vi "DG GUI Measurement setup.vi"(9 "DG measurement":T1={"Signal frequencies (Hz)"=[1000.0], "Signal amplitudes (V)"=[0.707], "Sampling frequencies (Hz)"=[10000000.0], "Record lengths (multiples of periods)"=[10000.0], "Calculate results"=FALSE, "Algorithm"="TWM-PJVSSubS", "TWM data directories"=[], "TWM data directories relative"=[], "PJVS frequencies (Hz)"=[1000.0], "PJVS reference voltages array of vector cluster"=[], "Requested PJVS steps"=[20], "Data folder"=path "", "Rs"=0, "Re"=0, "Settle down after PJVS change (s)"=1.0, "Switch position"=0.0, "PJVS amplitudes (Hz)"=[1000.0]} {"PJVS amplitudes (Hz)" format="%#_3p"; "PJVS reference voltages array of vector cluster"."PJVS reference voltages vector" format="%#_3p"; "PJVS frequencies (Hz)" format="%#_3p"; "Record lengths (multiples of periods)" format="%#_3p"; "Sampling frequencies (Hz)" format="%#_3p"; "Signal amplitudes (V)" format="%#_3p"; "Signal frequencies (Hz)" format="%#_3p"}) -> (3 "DG measurement out":T1={"Signal frequencies (Hz)"=[1000.0], "Signal amplitudes (V)"=[0.707], "Sampling frequencies (Hz)"=[10000000.0], "Record lengths (multiples of periods)"=[10000.0], "Calculate results"=FALSE, "Algorithm"="TWM-PJVSSubS", "TWM data directories"=[], "TWM data directories relative"=[], "PJVS frequencies (Hz)"=[1000.0], "PJVS reference voltages array of vector cluster"=[], "Requested PJVS steps"=[20], "Data folder"=path "", "Rs"=0, "Re"=0, "Settle down after PJVS change (s)"=1.0, "Switch position"=0.0, "PJVS amplitudes (Hz)"=[1000.0]} {"PJVS amplitudes (Hz)" format="%#_3p"; "PJVS reference voltages array of vector cluster"."PJVS reference voltages vector" format="%#_3p"; "PJVS frequencies (Hz)" format="%#_3p"; "Record lengths (multiples of periods)" format="%#_3p"; "Sampling frequencies (Hz)" format="%#_3p"; "Signal amplitudes (V)" format="%#_3p"; "Signal frequencies (Hz)" format="%#_3p"})   [LabVIEW 2020]
doc: "GUI to setup parameters of the digitizer gain calibration mesurement procedure."
uses:
  SS Measurement/Type definitions/SS measurement.ctl
  DG Measurement/DG measurement.ctl
  <vilib>/Utility/error.llb/Error Cluster From Error Code.vi
  <vilib>/ErrorRing/Error Ring.xnode
  external libraries/varilib/varilib.lvlib
panel:
  in  "Signal amplitude (V)":dbl=1.0 format="%#_13g"
  in  "Switch position":bool
  in  "Re":i32 min=0 step=1
  in  "Rs":i32 min=0 step=1
  out "No of samples":dbl format="%#_6p"
  out "Sampling time (s)":dbl
  out "DG error":string="!"
  out "Is coherent":string="!"
  in  "Data folder":path caption="Save data to folder:"
  in  "Requested PJVS steps":u32
  out "Requested PJVS steps out":u32[](array[numeric])
  in  "PJVS frequency (Hz)":dbl
  out "PJVS frequencies (Hz) out":dbl[](array[numeric])
  in  "Record length (multiple of period)":dbl
  out "SS measurement out":T2={"Signal frequencies (Hz)"=[1000.0], "Signal amplitudes (V)"=[0.707], "Sampling frequencies (Hz)"=[10000000.0], "Record lengths (multiples of periods)"=[10000.0], "Calculate results"=FALSE, "Algorithm"="TWM-WFFT", "TWM data directories"=[], "TWM data directories relative"=[], "Settle down after AC source change (s)"=1.0, "PJVS frequencies (Hz)"=[1000.0], "PJVS reference voltages array of vector cluster"=[{"PJVS reference voltages vector"=[]}], "Requested PJVS steps"=[20], "Measure CE"=FALSE, "Measure CE before"=FALSE, "Measure CE after"=FALSE, "Single point CE measurement"=FALSE, "original CE template path"=path "", "new CE template path before SS"=path "", "new CE template path before SS relative"=path "", "new CE template path after SS"=path "", "new CE template path after SS relative"=path "", "original CE fit path"=path "", "new CE fit path before SS"=path "", "new CE fit path before SS relative"=path "", "new CE fit path after SS"=path "", "new CE fit path after SS relative"=path "", "Measure digitizer gain"=FALSE, "Measure digitizer gain before"=FALSE, "Measure digitizer gain after"=FALSE, "Digitizer gain"=0.0, "Data folder"=path "", "FR fit path"=path "", "new FR fit path relative"=path "", "Rs"=0, "Re"=0, "SS measurement info files"=[]} {"PJVS reference voltages array of vector cluster"."PJVS reference voltages vector" format="%#_3p"; "PJVS frequencies (Hz)" format="%#_3p"; "Record lengths (multiples of periods)" format="%#_3p"; "Sampling frequencies (Hz)" format="%#_3p"; "Signal amplitudes (V)" format="%#_3p"; "Signal frequencies (Hz)" format="%#_3p"}
  in  "SS measurement":T2={"Signal frequencies (Hz)"=[1000.0], "Signal amplitudes (V)"=[0.707], "Sampling frequencies (Hz)"=[10000000.0], "Record lengths (multiples of periods)"=[10000.0], "Calculate results"=FALSE, "Algorithm"="TWM-WFFT", "TWM data directories"=[], "TWM data directories relative"=[], "Settle down after AC source change (s)"=1.0, "PJVS frequencies (Hz)"=[1000.0], "PJVS reference voltages array of vector cluster"=[{"PJVS reference voltages vector"=[]}], "Requested PJVS steps"=[20], "Measure CE"=FALSE, "Measure CE before"=FALSE, "Measure CE after"=FALSE, "Single point CE measurement"=FALSE, "original CE template path"=path "", "new CE template path before SS"=path "", "new CE template path before SS relative"=path "", "new CE template path after SS"=path "", "new CE template path after SS relative"=path "", "original CE fit path"=path "", "new CE fit path before SS"=path "", "new CE fit path before SS relative"=path "", "new CE fit path after SS"=path "", "new CE fit path after SS relative"=path "", "Measure digitizer gain"=FALSE, "Measure digitizer gain before"=FALSE, "Measure digitizer gain after"=FALSE, "Digitizer gain"=0.0, "Data folder"=path "", "FR fit path"=path "", "new FR fit path relative"=path "", "Rs"=0, "Re"=0, "SS measurement info files"=[]} {"PJVS reference voltages array of vector cluster"."PJVS reference voltages vector" format="%#_3p"; "PJVS frequencies (Hz)" format="%#_3p"; "Record lengths (multiples of periods)" format="%#_3p"; "Sampling frequencies (Hz)" format="%#_3p"; "Signal amplitudes (V)" format="%#_3p"; "Signal frequencies (Hz)" format="%#_3p"}
  in  "Calculate results":bool
  in  "Algorithm":string
  out "Signal amplitudes (V) out":dbl[](array[numeric])
  out "Record lengths (multiples of period)":dbl[](array[numeric])
  out "Sampling frequencies (Hz) out":dbl[](array[numeric])
  in  "Settle down after PJVS change (s)":dbl=1.0 format="%#_13g"
  in  "Sampling frequency (Hz)":dbl=10000000.0 format="%#_13p"
  in  "show connections":bool
  out "gui_elements":refnum<vi>[](array[refnum])
  in  "save_and_quit":bool
  in  "cancel":bool
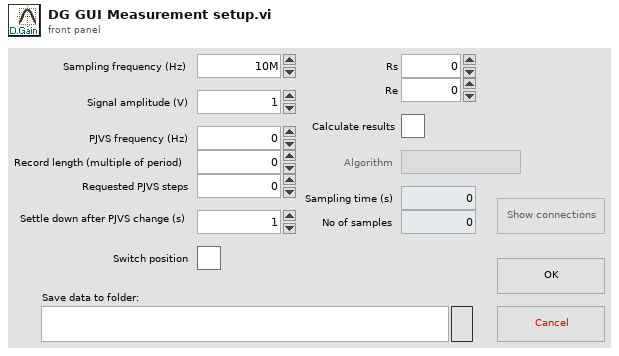
[diagram p1: front panel]
types:
  T1 = typedef "DG measurement.ctl" = cluster{"Signal frequencies (Hz)":dbl[], "Signal amplitudes (V)":dbl[], "Sampling frequencies (Hz)":dbl[], "Record lengths (multiples of periods)":dbl[], "Calculate results":bool, "Algorithm":string, "TWM data directories":path[], "TWM data directories relative":path[], "PJVS frequencies (Hz)":dbl[], "PJVS reference voltages array of vector cluster":cluster{"PJVS reference voltages vector":dbl[]}[], "Requested PJVS steps":u32[], "Data folder":path, "Rs":i32, "Re":i32, "Settle down after PJVS change (s)":dbl, "Switch position":dbl, "PJVS amplitudes (Hz)":dbl[]}
  T2 = typedef "SS measurement.ctl" = cluster{"Signal frequencies (Hz)":dbl[], "Signal amplitudes (V)":dbl[], "Sampling frequencies (Hz)":dbl[], "Record lengths (multiples of periods)":dbl[], "Calculate results":bool, "Algorithm":string, "TWM data directories":path[], "TWM data directories relative":path[], "Settle down after AC source change (s)":dbl, "PJVS frequencies (Hz)":dbl[], "PJVS reference voltages array of vector cluster":cluster{"PJVS reference voltages vector":dbl[]}[], "Requested PJVS steps":u32[], "Measure CE":bool, "Measure CE before":bool, "Measure CE after":bool, "Single point CE measurement":bool, "original CE template path":path, "new CE template path before SS":path, "new CE template path before SS relative":path, "new CE template path after SS":path, "new CE template path after SS relative":path, "original CE fit path":path, "new CE fit path before SS":path, "new CE fit path before SS relative":path, "new CE fit path after SS":path, "new CE fit path after SS relative":path, "Measure digitizer gain":bool, "Measure digitizer gain before":bool, "Measure digitizer gain after":bool, "Digitizer gain":dbl, "Data folder":path, "FR fit path":path, "new FR fit path relative":path, "Rs":i32, "Re":i32, "SS measurement info files":path[]}
  T3 = enum32{"Bad", "Idle", "Run top level", "Running"}
  T4 = cluster{"PJVS reference voltages vector":dbl[]}[]
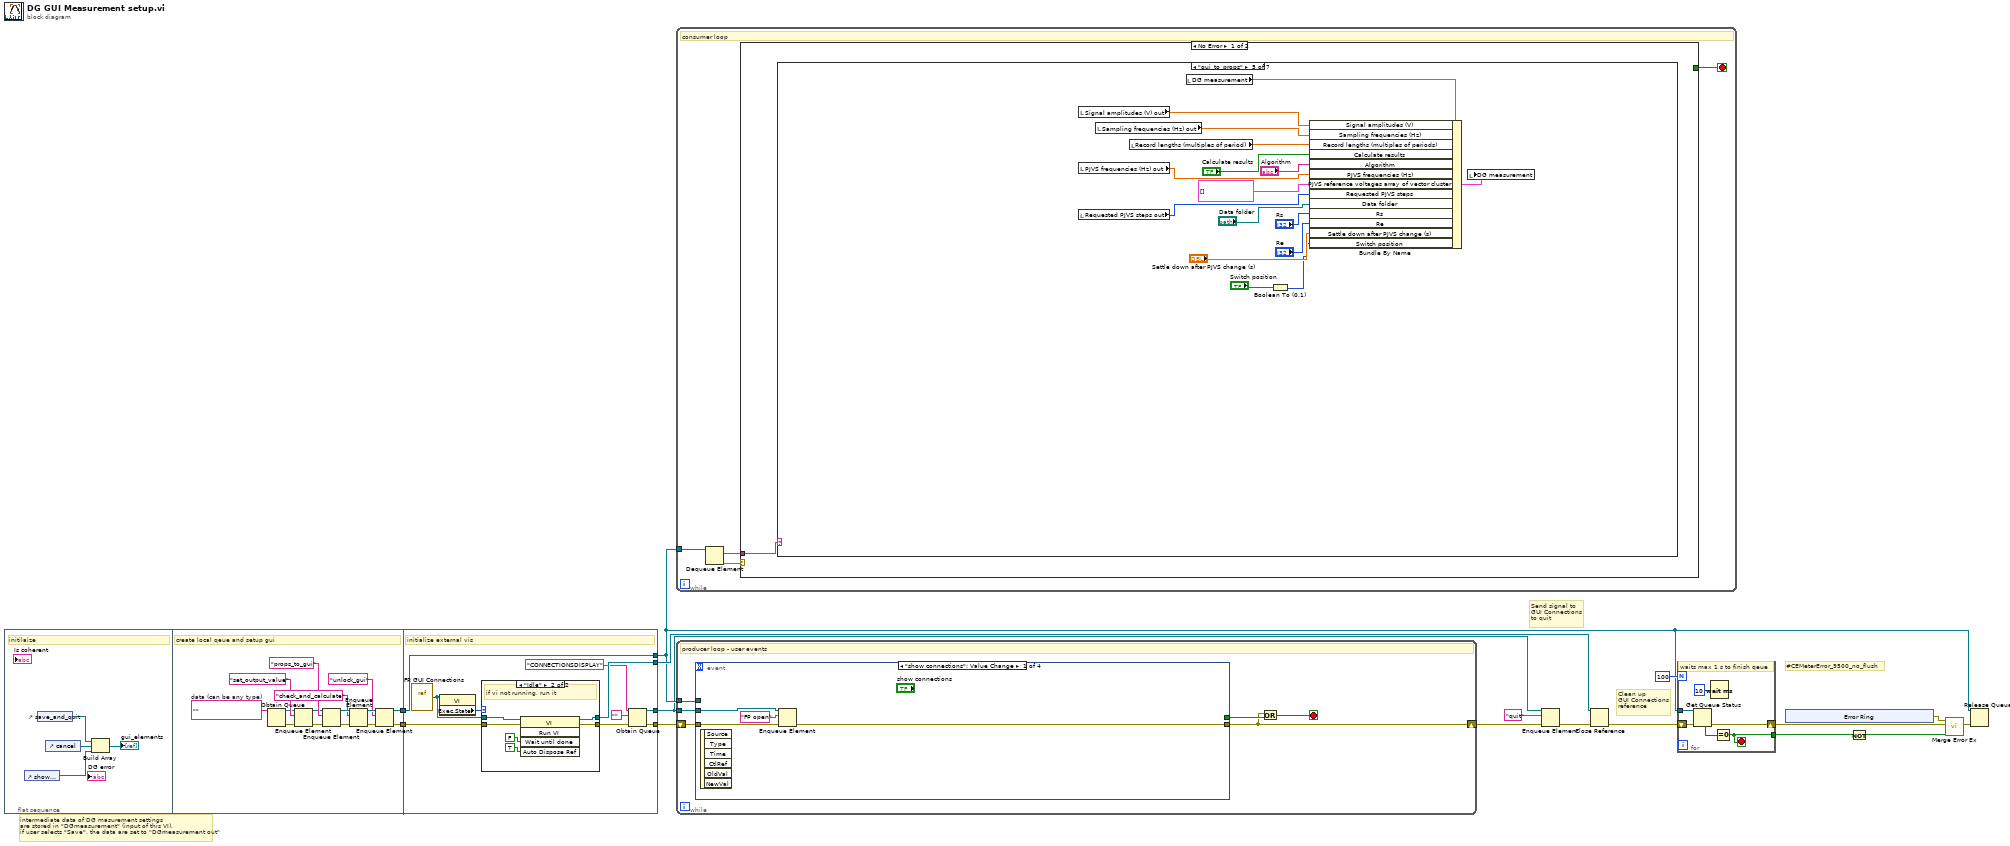
[diagram p0: block diagram]
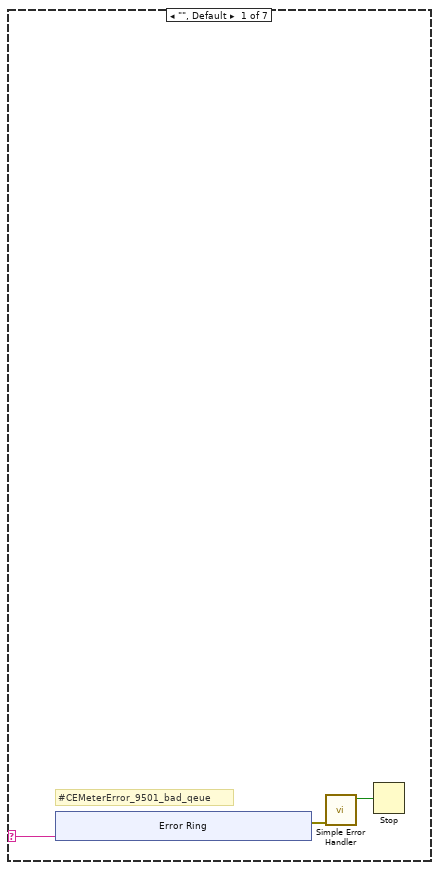
[diagram p3: hidden frame]
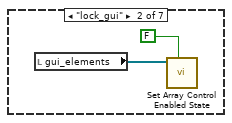
[diagram p4: hidden frame]
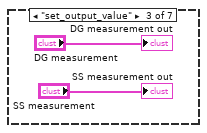
[diagram p5: hidden frame]
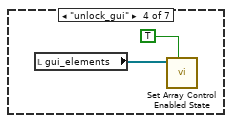
[diagram p6: hidden frame]
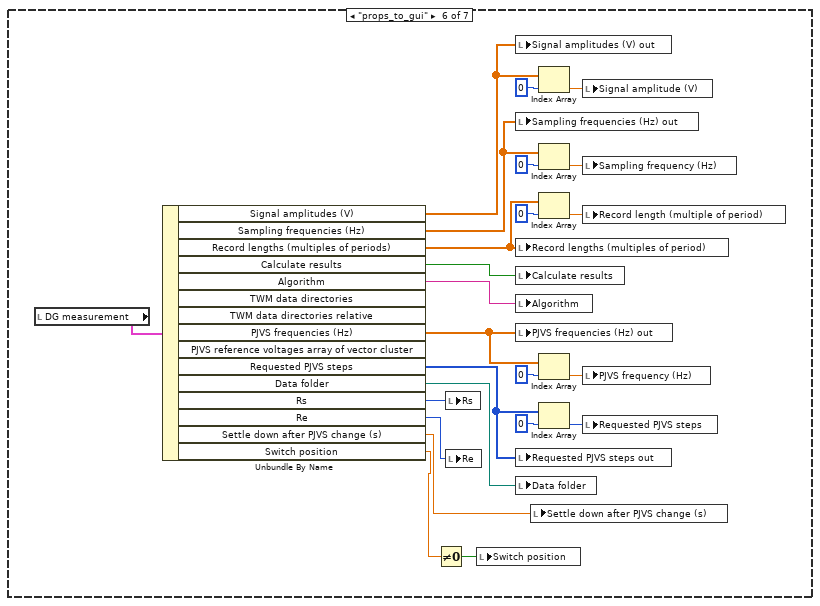
[diagram p7: hidden frame]
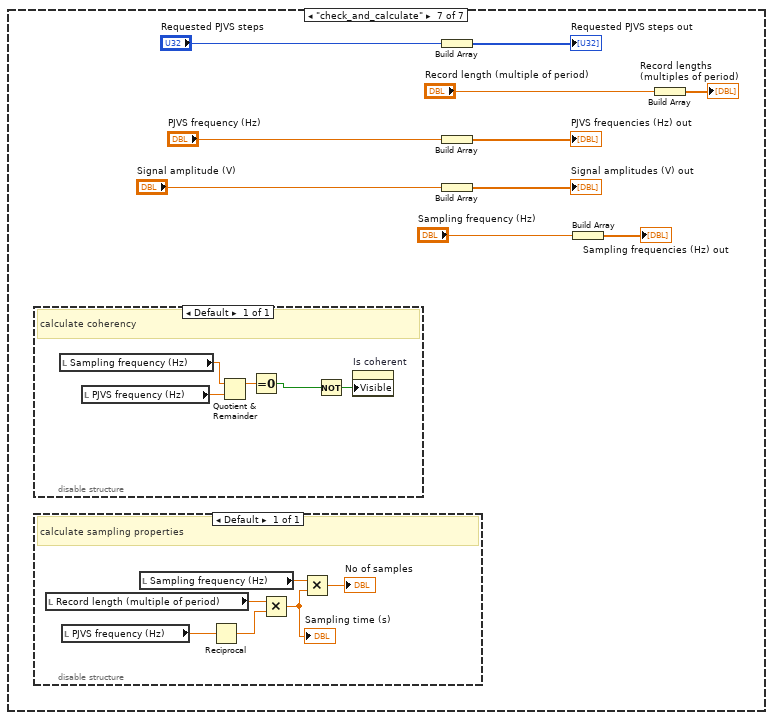
[diagram p8: hidden frame]
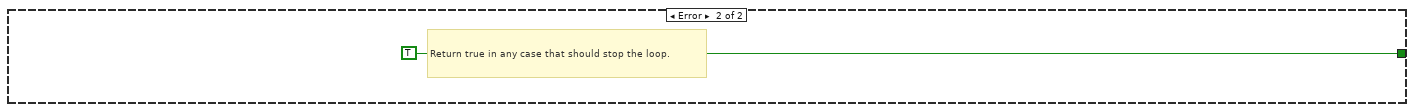
[diagram p9: hidden frame]
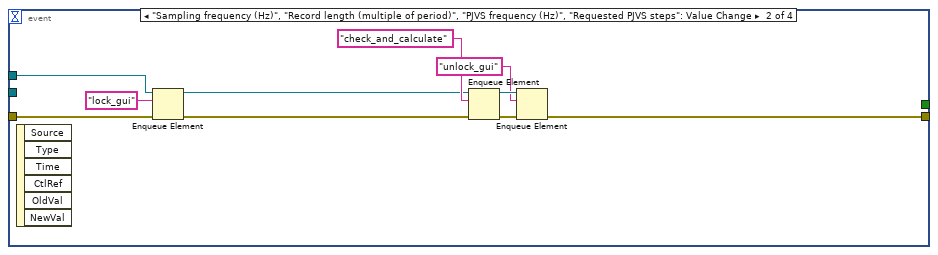
[diagram p10: hidden frame]
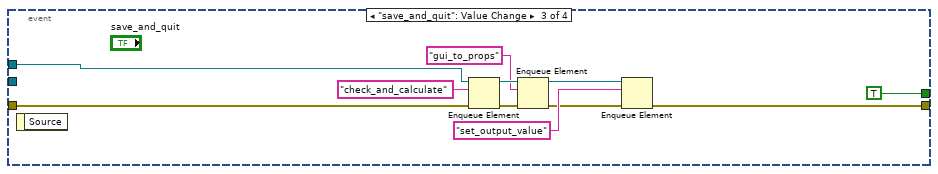
[diagram p11: hidden frame]
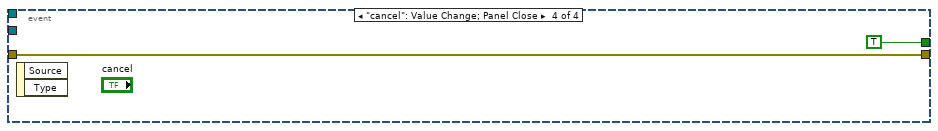
[diagram p12: hidden frame]
diagram:
  # "intermediate data of DG masurement settings\nare stored in \"DGmeasurement\" (input of this VI),\nif user selects \"Save\", the data are set to \"DGmeasurement out\""
  # "Send signal to\nGUI Connections\nto quit"
  # "Clean up\nGUI Connections\nreference"
  # "#CEMeterError_9500_no_flush"
  n1 = flat-sequence {
    tunnel: [w25] -> w9
    tunnel: [w24] -> w1
    tunnel: [w41] -> w10
    tunnel: [w45] -> w4
    tunnel: w9 -> [w44]
    tunnel: [w42] -> w3
    tunnel: [w43] -> w6
    tunnel: w1 -> [w45]
    frame #0 {
      # "initilaize"
      n2 = control-ref of="show connections"() -> (w17:refnum<vi>)
      n3 = control-ref of="save_and_quit"() -> (w20:refnum<vi>)
      n4 = control-ref of="cancel"() -> (w19:refnum<vi>)
      n5 = Build Array(w20, w19, w17) -> (→"gui_elements":refnum<vi>[])
    }
    frame #1 {
      w34 = ""  # data (can be any type)
      # "create local qeue and setup gui"
      n6 = Obtain Queue(element data type=w34) -> (queue out=w27:refnum<queue>, error out=w26:errorcluster)  [unwired: 4 in, 1 out]
      n7 = Enqueue Element(queue=w27, element="set_output_value", error in (no error)=w26) -> (queue out=w29:refnum<queue>, error out=w28:errorcluster)  [unwired: 1 in, 1 out]
      n8 = Enqueue Element(queue=w29, element="props_to_gui", error in (no error)=w28) -> (queue out=w32:refnum<queue>, error out=w33:errorcluster)  [unwired: 1 in, 1 out]
      n9 = Enqueue Element(queue=w32, element="check_and_calculate", error in (no error)=w33) -> (queue out=w23:refnum<queue>, error out=w22:errorcluster)  [unwired: 1 in, 1 out]
      n10 = Enqueue Element(queue=w23, element="unlock_gui", error in (no error)=w22) -> (queue out=w24:refnum<queue>, error out=w25:errorcluster)  [unwired: 1 in, 1 out]
    }
    frame #2 {
      # "initialize external vis"
      n11 = vi-ref "FR GUI Connections.vi"() -> (w39:refnum<vi>)
      n12 = property class="VI"(reference=w39) -> ("Exec.State"=w40:T3)  [unwired: 1 in, 2 out]
      n13 = case shown="\"Idle\"" w40 {
        tunnel: [w46 w53] -> w36
        tunnel: w44 -> [w46 w50]
        tunnel: [w47 w49] -> w43
        tunnel: w39 -> [w47 w48]
        frame "Bad", Default {
        }
        frame "Idle" {
          # "if vi not running, run it"
          n14 = invoke class="VI" method="Run VI"(reference=w48, error in=w50, "Wait until done"=FALSE ("Wait Until Done"), "Auto Dispose Ref"=TRUE ("Wait Until Done")) -> (reference out=w49:refnum<vi>, error out=w53:errorcluster)  [unwired: 1 in, 3 out]
        }
      }
      n15 = Obtain Queue(name (unnamed)="CONNECTIONSDISPLAY", element data type="", error in (no error)=w36) -> (queue out=w42:refnum<queue>, error out=w41:errorcluster)  [unwired: 2 in, 1 out]
    }
  }
  n16 = while {
    tunnel: w4 -> [w57]
    stop <- w54 stop-if-true
    # "consumer loop"
    n17 = Dequeue Element(queue=w57) -> (element=w55:string, error out=w56:errorcluster)  [unwired: 2 in, 2 out]
    n18 = case shown="No Error" w56 {
      tunnel: w55 -> [w58 _]
      tunnel: [_ TRUE] -> w54
      frame No Error {
        n19 = case shown="\"gui_to_props\"" w58 {
          selector: w58 -> [w59 _ _ _ _ _ _]
          frame "", Default {
            # "#CEMeterError_9501_bad_qeue"
            n20 = xnode "Error Ring"("parameter 0"=w59) -> ("error out"=w61:errorcluster)
            n21 = call <vilib>:"Simple Error Handler.vi"("error in (no error)"=w61) -> ("error?"=w60:bool)  [unwired: 4 in, 4 out]
            n22 = Stop(stop? (T)=w60) -> ()
          }
          frame "lock_gui" {
            n23 = local read "gui_elements"() -> (w70:refnum<vi>[])
            n24 = call "Set Array Control Enabled State.vi"("enabled (T)"=FALSE, "reference array in"=w70) -> ()  [unwired: 8 in, 2 out]
          }
          frame "set_output_value" {
            "SS measurement out" <- "SS measurement"
            "DG measurement out" <- "DG measurement"
          }
          frame "unlock_gui" {
            n25 = local read "gui_elements"() -> (w74:refnum<vi>[])
            n26 = call "Set Array Control Enabled State.vi"("enabled (T)"=TRUE, "reference array in"=w74) -> ()  [unwired: 8 in, 2 out]
          }
          frame "gui_to_props" {
            n27 = local read "Signal amplitudes (V) out"() -> (w86:dbl[])
            n28 = local read "PJVS frequencies (Hz) out"() -> (w81:dbl[])
            n29 = local read "Requested PJVS steps out"() -> (w79:u32[])
            n30 = local read "Sampling frequencies (Hz) out"() -> (w85:dbl[])
            n31 = local read "Record lengths (multiples of period)"() -> (w84:dbl[])
            n32 = local read "DG measurement"() -> (w90:T1)
            n33 = Boolean To (0,1)(Boolean="Switch position") -> (0, 1=w76:i16)
            n34 = Bundle By Name(cluster=w90, "Signal amplitudes (V)"=w86, "Sampling frequencies (Hz)"=w85, "Record lengths (multiples of periods)"=w84, "Calculate results"="Calculate results", "Algorithm"="Algorithm", "PJVS frequencies (Hz)"=w81, "PJVS reference voltages array of vector cluster"=T4 [], "Requested PJVS steps"=w79, "Data folder"="Data folder", "Rs"="Rs", "Re"="Re", "Settle down after PJVS change (s)"="Settle down after PJVS change (s)", "Switch position"=w76) -> (w89:T1)
            n35 = local write "DG measurement"(w89) -> ()
          }
          frame "props_to_gui" {
            n36 = local read "DG measurement"() -> (w104:T1)
            n37 = Unbundle By Name(w104) -> ("Signal amplitudes (V)"=w93:dbl[], "Sampling frequencies (Hz)"=w94:dbl[], "Record lengths (multiples of periods)"=w95:dbl[], "Calculate results"=w96:bool, "Algorithm"=w97:string, "PJVS frequencies (Hz)"=w98:dbl[], "Requested PJVS steps"=w99:u32[], "Data folder"=w100:path, "Rs"=w101:i32, "Re"=w102:i32, "Settle down after PJVS change (s)"=w103:dbl, "Switch position"=w92:dbl)  [unwired: 3 out]
            n38 = Not Equal To 0?(x=w92) -> (x != 0?=w91:bool)
            n39 = local write "Rs"(w101) -> ()
            n40 = local write "Re"(w102) -> ()
            n41 = local write "Switch position"(w91) -> ()
            n42 = local write "Signal amplitudes (V) out"(w93) -> ()
            n43 = local write "Sampling frequencies (Hz) out"(w94) -> ()
            n44 = local write "Record lengths (multiples of period)"(w95) -> ()
            n45 = local write "Calculate results"(w96) -> ()
            n46 = local write "Algorithm"(w97) -> ()
            n47 = local write "PJVS frequencies (Hz) out"(w98) -> ()
            n48 = local write "Requested PJVS steps out"(w99) -> ()
            n49 = local write "Data folder"(w100) -> ()
            n50 = local write "Settle down after PJVS change (s)"(w103) -> ()
            n51 = Index Array(array=w93, index=0) -> (element=w114:dbl)
            n52 = Index Array(array=w94, index=0) -> (element=w111:dbl)
            n53 = Index Array(array=w95, index=0) -> (element=w109:dbl)
            n54 = Index Array(array=w98, index=0) -> (element=w105:dbl)
            n55 = Index Array(array=w99, index=0) -> (element=w106:u32)
            n56 = local write "Signal amplitude (V)"(w114) -> ()
            n57 = local write "Sampling frequency (Hz)"(w111) -> ()
            n58 = local write "Record length (multiple of period)"(w109) -> ()
            n59 = local write "PJVS frequency (Hz)"(w105) -> ()
            n60 = local write "Requested PJVS steps"(w106) -> ()
          }
          frame "check_and_calculate" {
            n61 = disable-structure shown="Default" {
              frame Enabled {
                # "calculate coherency"
                n62 = local read "Sampling frequency (Hz)"() -> (w135:dbl)
                n63 = local read "PJVS frequency (Hz)"() -> (w134:dbl)
                n64 = Quotient & Remainder(x=w135, y=w134) -> (x-y*floor(x/y)=w133:dbl)  [unwired: 1 out]
                n65 = Equal To 0?(x=w133) -> (x = 0?=w131:bool)
                n66 = Not(x=w131) -> (.not. x?=w132:bool)
                n67 = property on="Is coherent" class="Str"("Visible"=w132) -> ()  [unwired: 2 in, 2 out]
              }
            }
            n68 = disable-structure shown="Default" {
              frame Enabled {
                # "calculate sampling properties"
                n69 = local read "Record length (multiple of period)"() -> (w128:dbl)
                n70 = local read "PJVS frequency (Hz)"() -> (w130:dbl)
                n71 = local read "Sampling frequency (Hz)"() -> (w127:dbl)
                n72 = Reciprocal(x=w130) -> (1/x=w129:dbl)
                n73 = Multiply(x=w128, y=w129) -> (x*y=w125:dbl)
                "Sampling time (s)" <- w125
                n74 = Multiply(x=w127, y=w125) -> (x*y=→"No of samples":dbl)
              }
            }
            n75 = Build Array("Requested PJVS steps") -> (→"Requested PJVS steps out":u32[])
            n76 = Build Array("PJVS frequency (Hz)") -> (→"PJVS frequencies (Hz) out":dbl[])
            n77 = Build Array("Signal amplitude (V)") -> (→"Signal amplitudes (V) out":dbl[])
            n78 = Build Array("Sampling frequency (Hz)") -> (→"Sampling frequencies (Hz) out":dbl[])
            n79 = Build Array("Record length (multiple of period)") -> (→"Record lengths (multiples of period)":dbl[])
          }
        }
      }
      frame Error {
        # "Return true in any case that should stop the loop."
      }
    }
  }
  n80 = while {
    shift-right: [w138] -> w5
    shift-left: w10 -> [w141]
    tunnel: w4 -> [w142]
    tunnel: w3 -> [w137]
    stop <- w139 stop-if-true
    # "producer loop - user events"
    n81 = event shown="[0] \"show connections\": Value Change" {
      selector: _ -> [_ _ _ _]
      dyn-events: _ -> [_ _ _ _]
      timeout: _ -> [_ _ _ _]
      tunnel: w142 -> [_ w155 w166 _]
      tunnel: w141 -> [w145 w148 w165 w168]
      tunnel: [w144 w147 w164 w168] -> w138
      tunnel: [_ _ TRUE ("cancel") TRUE ("cancel")] -> w140
      tunnel: w137 -> [w143 _ _ _]
      event "show connections": Value Change {
        n82 = event-data() -> ()  [unwired: 1 in, 6 out]
        n83 = Enqueue Element(queue=w143, element="FP open", error in (no error)=w145) -> (error out=w144:errorcluster)  [unwired: 1 in, 2 out]
      }
      event "Sampling frequency (Hz)", "Record length (multiple of period)", "PJVS frequency (Hz)", "Requested PJVS steps": Value Change {
        n84 = event-data() -> ()  [unwired: 1 in, 6 out]
        n85 = Enqueue Element(queue=w155, element="lock_gui", error in (no error)=w148) -> (queue out=w154:refnum<queue>, error out=w149:errorcluster)  [unwired: 1 in, 1 out]
        n86 = Enqueue Element(queue=w154, element="check_and_calculate", error in (no error)=w149) -> (queue out=w153:refnum<queue>, error out=w150:errorcluster)  [unwired: 1 in, 1 out]
        n87 = Enqueue Element(queue=w153, element="unlock_gui", error in (no error)=w150) -> (error out=w147:errorcluster)  [unwired: 1 in, 2 out]
      }
      event "save_and_quit": Value Change {
        n88 = event-data() -> ()  [unwired: 1 in, 1 out]
        n89 = Enqueue Element(queue=w166, element="check_and_calculate", error in (no error)=w165) -> (queue out=w161:refnum<queue>, error out=w162:errorcluster)  [unwired: 1 in, 1 out]
        n90 = Enqueue Element(queue=w161, element="gui_to_props", error in (no error)=w162) -> (queue out=w160:refnum<queue>, error out=w159:errorcluster)  [unwired: 1 in, 1 out]
        n91 = Enqueue Element(queue=w160, element="set_output_value", error in (no error)=w159) -> (error out=w164:errorcluster)  [unwired: 1 in, 2 out]
      }
      event "cancel": Value Change; Panel Close {
        n92 = event-data() -> ()  [unwired: 1 in, 2 out]
      }
    }
    n93 = Or(x=w138, y=w140) -> (x .or. y?=w139:bool)
  }
  n94 = Enqueue Element(queue=w3, element="quit", error in (no error)=w5) -> (error out=w8:errorcluster)  [unwired: 1 in, 2 out]
  n95 = Close Reference(reference=w6, error in (no error)=w8) -> (error out=w2:errorcluster)
  n96 = for {
    N: 100 -> [_]
    tunnel: w4 -> [w175]
    shift-right: [w173] -> w13
    shift-left: w2 -> [w174]
    tunnel: [w170] -> w11
    stop <- w170 stop-if-true
    # "waits max 1 s to finish qeue"
    n97 = Get Queue Status(queue=w175, error in (no error)=w174) -> (error out=w173:errorcluster, # elements in queue=w171:i32)  [unwired: 1 in, 6 out]
    n98 = Wait (ms)(milliseconds to wait=u32 10) -> ()  [unwired: 1 out]
    n99 = Equal To 0?(x=w171) -> (x = 0?=w170:bool)
  }
  n100 = xnode "Error Ring"() -> ("error out"=w14:errorcluster)
  n101 = Not(x=w11) -> (.not. x?=w15:bool)
  n102 = call "Merge Error Ex.vi"("Is error? (False)"=w15, "main error in (no error)"=w13, "second error in"=w14) -> ("error out"=w12:errorcluster)  [unwired: 8 in]
  n103 = Release Queue(queue=w4, error in (no error)=w12) -> ()  [unwired: 1 in, 3 out]
